vi "DMAC String to DMAC U8.vi"(5 "DMAC String":string) -> (2 "DestinationMACAddress":u8[](array[numeric])=[3, 0, 94, 160, 3, 233] format="%02x")   [LabVIEW 2021, in "Networking_CIF_U.lvlib"]
uses:
  Networking_CIF_U.lvlib
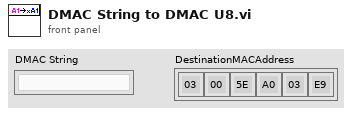
[diagram p1: front panel]
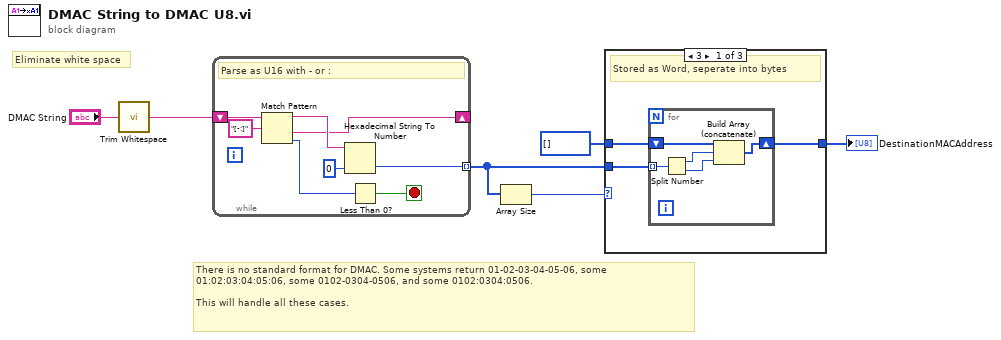
[diagram p0: block diagram]
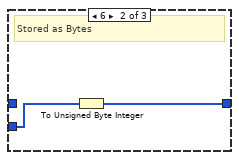
[diagram p2: hidden frame]
diagram:
  # "Eliminate white space"
  # "There is no standard format for DMAC. Some systems return 01-02-03-04-05-06, some 01:02:03:04:05:06, some 0102-0304-0506, and some 0102:0304:0506. \n\nThis will handle all these cases."
  n1 = call <vilib>:"Trim Whitespace.vi"("string"="DMAC String") -> ("trimmed string"=w5:string)  [unwired: 1 in]
  n2 = while {
    shift-right: [w8] -> _
    shift-left: w5 -> [w13]
    tunnel: [w11] -> w3 mode=indexing
    stop <- w10 stop-if-true
    # "Parse as U16 with - or :"
    n3 = Match Pattern(string=w13, regular expression="[-:]") -> (before substring=w12:string, after substring=w8:string, offset past match=w9:i32)  [unwired: 1 in, 1 out]
    n4 = Hexadecimal String To Number(string=w12, default (0uL)=u16 0 ("default (0 U32)")) -> (number=w11:u16)  [unwired: 1 in, 1 out]
    n5 = Less Than 0?(x=w9) -> (x < 0?=w10:bool)
  }
  n6 = Array Size(array=w3) -> (size(s)=w4:i32)
  n7 = case shown="3" w4 {
    tunnel: w3 -> [w17 w24 _]
    tunnel: u8[] [] -> [w16 _ w25]
    tunnel: [w15 w23 w25] -> w1
    frame 3 {
      # "Stored as Word, seperate into bytes"
      n8 = for {
        tunnel: w17 -> [w21] mode=indexing
        shift-right: [w18] -> w15
        shift-left: w16 -> [w22]
        n9 = Split Number(x=w21) -> (hi(x)=w20:u8, lo(x)=w19:u8)
        n10 = Build Array (concatenate)(w22, w20, w19) -> (w18:u8[])
      }
    }
    frame 6 {
      # "Stored as Bytes"
      n11 = To Unsigned Byte Integer(number=w24) -> (unsigned 8bit integer=w23:u8[])
    }
    frame 0, Default {
      # "Could set error code here"
      # "Incorrect length, Unable to parse"
    }
  }
  "DestinationMACAddress" <- w1
